vi "ReadXML_TCP.vi"(3 "error in":errorcluster, 4 "timeout ms (3000)":i32=3000, 5 "connection ID in":refnum<k5>) -> (0 "error out":errorcluster, 1 "data out":string, 2 "connection ID out":refnum<k5>)   [LabVIEW 2016]
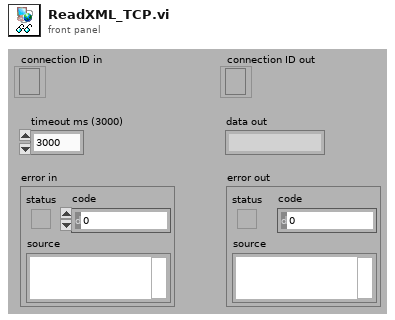
[diagram p1: front panel]
types:
  T1 = enum16{"Standard", "Buffered", "CRLF", "Immediate"}
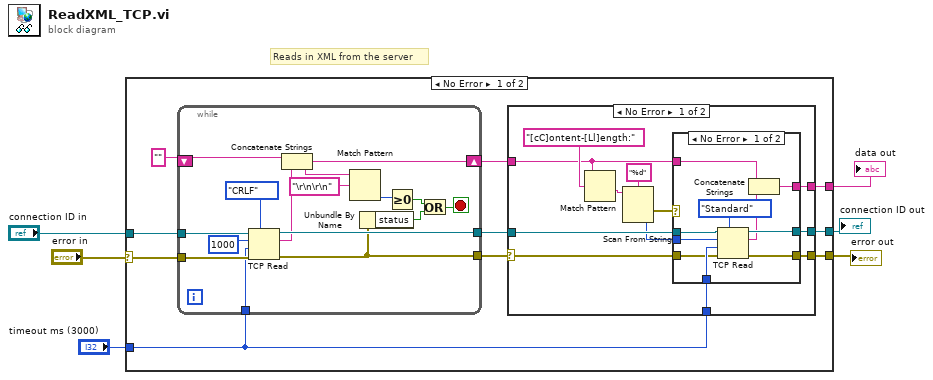
[diagram p0: block diagram]
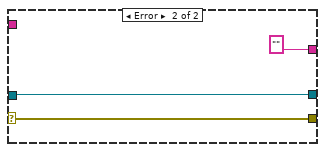
[diagram p3: hidden frame]
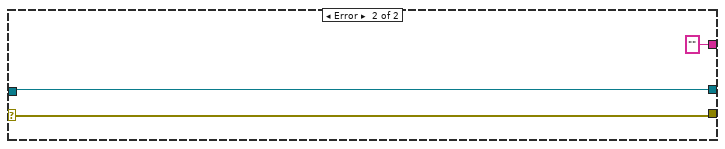
[diagram p4: hidden frame]
diagram:
  # "Reads in XML from the server"
  n1 = case shown="No Error" "error in" {
    selector: "error in" -> [w7 w62]
    tunnel: "timeout ms (3000)" -> [w16 _]
    tunnel: [w15 "" ("data out")] -> w5
    tunnel: [w14 w61] -> w4
    tunnel: [w13 w62] -> w3
    tunnel: "connection ID in" -> [w9 w61]
    frame No Error {
      n2 = while {
        tunnel: [w59] -> w12
        tunnel: w9 -> [w58]
        tunnel: w7 -> [w57]
        tunnel: [w45] -> w8
        shift-right: [w52] -> w11
        shift-left: "" -> [w53]
        tunnel: w16 -> [w46]
        stop <- w47 stop-if-true
        n3 = TCP Read(connection ID=w58, bytes to read=1000, error in (no error)=w57, 7:T1."CRLF" ("mode (standard)"), 9:w46) -> (connection ID out=w59:refnum<k5>, data out=w54:string, error out=w45:errorcluster)
        n4 = Concatenate Strings(w53, w54) -> (w52:string)
        n5 = Match Pattern(string=w52, regular expression="\r\n\r\n") -> (offset past match=w50:i32)  [unwired: 1 in, 3 out]
        n6 = Unbundle By Name(w45) -> ("status"=w48:bool)
        n7 = Greater Or Equal To 0?(x=w50) -> (x >= 0?=w49:bool)
        n8 = Or(x=w49, y=w48) -> (x .or. y?=w47:bool)
      }
      n9 = case shown="No Error" w8 {
        selector: w8 -> [w17 w42]
        tunnel: w16 -> [w28 _]
        tunnel: [w19 "" ("data out")] -> w15
        tunnel: [w27 w44] -> w14
        tunnel: [w26 w42] -> w13
        tunnel: w12 -> [w25 w44]
        tunnel: w11 -> [w20 _]
        frame No Error {
          n10 = Match Pattern(string=w20, regular expression="[cC]ontent-[Ll]ength:") -> (after substring=w22:string)  [unwired: 1 in, 3 out]
          n11 = Scan From String(format string="%d", input string=w22) -> (error out=w18:errorcluster, output 1=w24:i32)  [unwired: 3 in, 2 out]
          n12 = case shown="No Error" w18 {
            tunnel: w28 -> [w38 _]
            tunnel: [w37 w39] -> w27
            tunnel: [w36 w40] -> w26
            tunnel: w17 -> [w35 w40]
            tunnel: w25 -> [w34 w39]
            tunnel: w24 -> [w32 _]
            tunnel: w20 -> [w31 w41]
            tunnel: [w29 w41] -> w19
            frame No Error {
              n13 = TCP Read(connection ID=w34, bytes to read=w32, error in (no error)=w35, 7:T1."Standard" ("mode (standard)"), 9:w38) -> (connection ID out=w37:refnum<k5>, data out=w30:string, error out=w36:errorcluster)
              n14 = Concatenate Strings(w31, w30) -> (w29:string)
            }
            frame Error {
            }
          }
        }
        frame Error {
        }
      }
    }
    frame Error {
    }
  }
  "data out" <- w5
  "connection ID out" <- w4
  "error out" <- w3
